vi "HAL Camera specifications globals.vi"() -> ()   [LabVIEW 2016]
panel:
  in  "Allowed camera models":string[](array[string])
  in  "Shift settings table":T1(array[cluster])=[{"Adc Channel"=0, "H Shift Setting"=0, "EM on?"=TRUE}, {"Adc Channel"=0, "H Shift Setting"=1, "EM on?"=TRUE}, {"Adc Channel"=0, "H Shift Setting"=2, "EM on?"=TRUE}, {"Adc Channel"=0, "H Shift Setting"=3, "EM on?"=TRUE}, {"Adc Channel"=0, "H Shift Setting"=0, "EM on?"=FALSE}, {"Adc Channel"=0, "H Shift Setting"=1, "EM on?"=FALSE}]
  in  "Camera Name":string="Andor iXon  Ultra 1024"
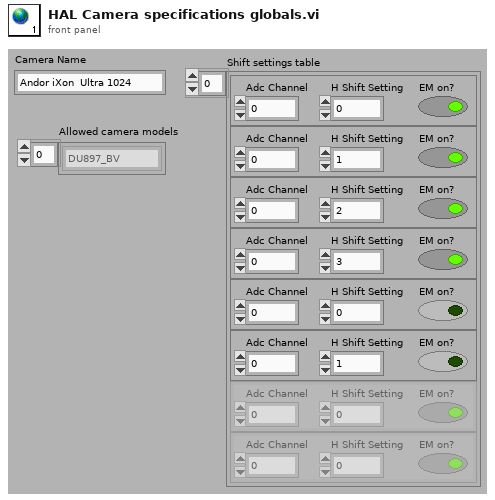
[diagram p1: front panel]
types:
  T1 = cluster{"Adc Channel":i32, "H Shift Setting":i32, "EM on?":bool}[]
diagram:
